vi "PH_Switch.set i Attr.vi"(0 "VI in":refnum<vi>, 5 "error in (no error)":errorcluster) -> (14 "VI out":refnum<vi>, 16 "i Attribute":T1 {"Status Switch State" items=["no info", "off/false/out", "on/true/in", "Failure", "Alarm", "Status 1", "Status 2", "Status 3"]; "Status false" items=["no info", "off/false/out", "on/true/in", "Failure", "Alarm", "Status 1", "Status 2", "Status 3"]; "Status true" items=["no info", "off/false/out", "on/true/in", "Failure", "Alarm", "Status 1", "Status 2", "Status 3"]}, 19 "error out":errorcluster)   [LabVIEW 2014, in "PH_Switch.lvlib"]
uses:
  PH_Switch.lvlib
  PH_Switch.i attribute.ctl
  PH_Switch.GUI Refs.ctl
  PH_StatusHandler/PH_StatusHandler.Status.ctl
  CSCore/CSSystem/CSSystemLib/CSSystemLib.lvlib
  PH_StatusHandler/PH_StatusHandler.lvlib
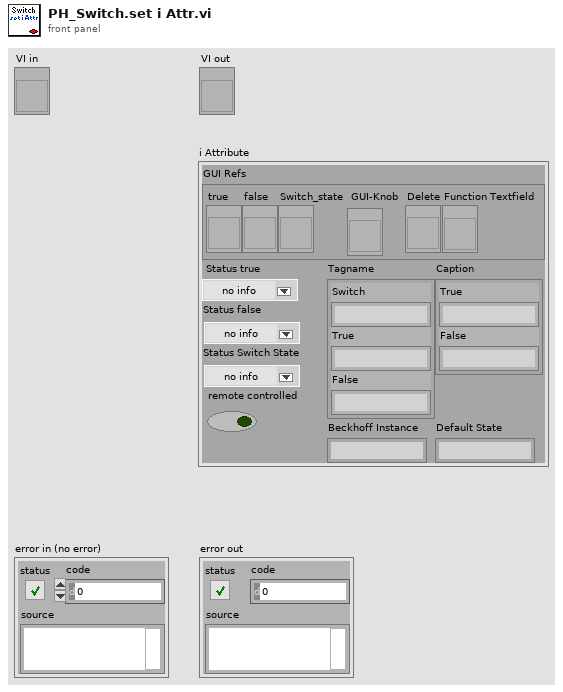
[diagram p1: front panel]
types:
  T1 = typedef "PH_Switch.lvlib/PH_Switch.i attribute.ctl" = cluster{"GUI Refs":T2, "Status true":T3, "Status false":T3, "Status Switch State":T3, "remote controlled":bool, "Tagname":cluster{"Switch":string, "True":string, "False":string}, "Beckhoff Instance":string, "Caption":cluster{"True":string, "False":string}, "Default State":string}
  T2 = typedef "PH_Switch.lvlib/PH_Switch.GUI Refs.ctl" = cluster{"true":refnum<vi>, "false":refnum<vi>, "Switch_state":refnum<vi>, "GUI-Knob":refnum<vi>, "Delete":refnum<vi>, "Function Textfield":refnum<vi>}
  T3 = typedef "PH_StatusHandler.lvlib/PH_StatusHandler.Status.ctl" = i16
  T4 = cluster{"Switch":string, "True":string, "False":string}
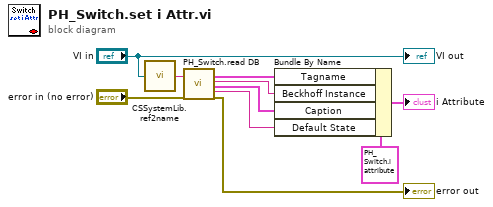
[diagram p0: block diagram]
diagram:
  n1 = call "CSSystemLib.ref2name.vi"("obj refnum"="VI in") -> ("name"=w3:string)
  n2 = call "PH_Switch.read DB.vi"("DB Entry to read"=w3, "error in (no error)"="error in (no error)") -> ("Tagnames"=w7:T4, "Beckhoff Instance"=w6:string, "Captions"=w5:cluster{"True":string, "False":string}, "Default Value"=w4:string, "error out"=→"error out":errorcluster)  [unwired: 13 in]
  n3 = Bundle By Name(cluster=T1 {"GUI Refs"={"true"=refnum, "false"=refnum, "Switch_state"=refnum, "GUI-Knob"=refnum, "Delete"=refnum, "Function Textfield"=refnum}, "Status true"=0, "Status false"=0, "Status Switch State"=0, "remote controlled"=FALSE, "Tagname"={"Switch"="N/A", "True"="N/A", "False"="N/A"}, "Beckhoff Instance"="N/A", "Caption"={"True"="", "False"=""}, "Default State"="N/A"} ("CLASS.i attribute"), "Tagname"=w7, "Beckhoff Instance"=w6, "Caption"=w5, "Default State"=w4) -> (→"i Attribute":T1)
  "VI out" <- "VI in"
